vi "Line.vi"(8 "Length":dbl, 9 "ContPow":T5, 10 "Y":dbl, 11 "X":dbl) -> (3 "PathSupreme":T1)   [LabVIEW 2014]
uses:
  TypeDefs/PowerSpeed.ctl
  TypeDefs/PathSupreme.ctl
  PSup2SCAN/Sub/VelocityProfile.ctl
  PSup2SCAN/Sub/PathCut.ctl
  PSup2SCAN/Sub/Segment.ctl
  TypeDefs/Point2DwSlope.ctl
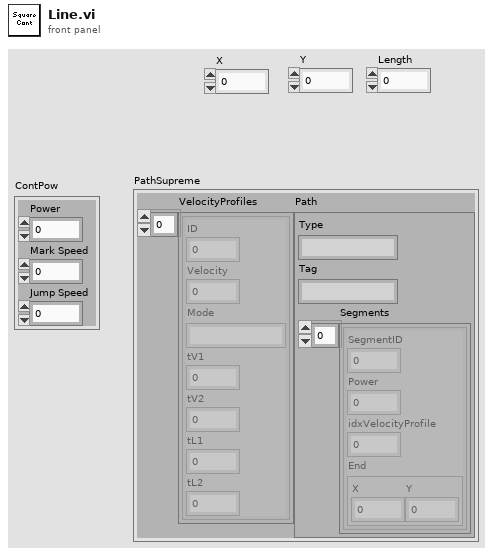
[diagram p1: front panel]
types:
  T1 = typedef "PathSupreme.ctl" = cluster{"VelocityProfiles":T2[], "Path":T3}
  T2 = typedef "VelocityProfile.ctl" = cluster{"ID":u32, "Velocity":dbl, "Mode":string, "tV1":u32, "tV2":u32, "tL1":u32, "tL2":u32}
  T3 = typedef "PathCut.ctl" = cluster{"Type":string, "Tag":string, "Segments":T4[]}
  T4 = typedef "Segment.ctl" = cluster{"SegmentID":u16, "Power":sgl, "idxVelocityProfile":u16, "End":cluster{"X":sgl, "Y":sgl}}
  T5 = typedef "PowerSpeed.ctl" = cluster{"Power":dbl, "Mark Speed":dbl, "Jump Speed":dbl}
  T6 = typedef "Point2DwSlope.ctl" = cluster{"X":sgl, "Y":sgl, "Slope":dbl}
  T7 = cluster{"VertexArray":T6[], "OnOffAr":enum16{"On", "Off"}[]}
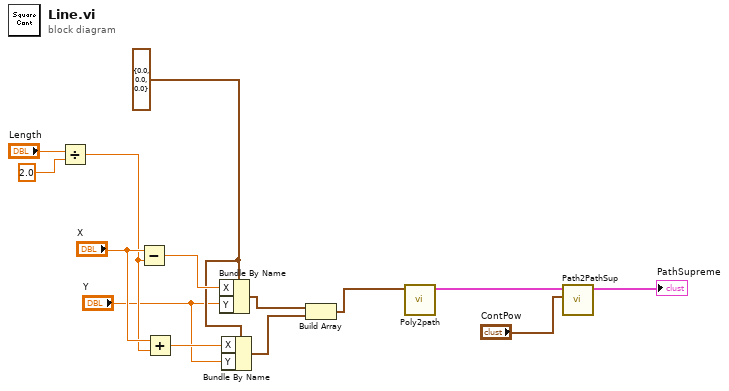
[diagram p0: block diagram]
diagram:
  w8 = T6 {"X"=0.0, "Y"=0.0, "Slope"=0.0} ("Point2D")
  n1 = Divide(x="Length", y=2.0) -> (x/y=w6:dbl)
  n2 = Subtract(x="X", y=w6) -> (x-y=w9:dbl)
  n3 = Add(x="X", y=w6) -> (x+y=w5:dbl)
  n4 = Bundle By Name(cluster=w8, "X"=w9, "Y"="Y") -> (w3:T6)
  n5 = Bundle By Name(cluster=w8, "X"=w5, "Y"="Y") -> (w2:T6)
  n6 = Build Array(w3, w2) -> (w1:T6[])
  n7 = call "Poly2path.vi"("VertexArray"=w1) -> ("Path"=w12:T7)  [unwired: 10 in]
  n8 = call "Path2PathSup.vi"("PowerSpeed"="ContPow", "Combined"=w12) -> ("PathSupreme"=→"PathSupreme":T1)  [unwired: 9 in]
